vi "Direttore.vi"() -> ()   [LabVIEW 2012]
uses:
  <vilib>/Platform/TimedLoop/XDataNode/timing_clust.ctl
  <vilib>/Platform/TimedLoop/XDataNode/nitl_modes.ctl
  <vilib>/Platform/TimedLoop/XDataNode/wakeup.ctl
  <vilib>/FPGAPlugInAG/PCIe-7852R/niLvFpga_Open_PCIe-7852R.vi
  <vilib>/rvi/interface/common/dynamic/niFpgaDynamicAddResources.vi
  <vilib>/FPGAPlugInAG/Dynamic/niLvFpga_Run_Dynamic.vi
  <vilib>/Utility/error.llb/Error Cluster From Error Code.vi
  <vilib>/rvi/errors/niLvFpgaAdjustHostInterfaceError.vi
  <vilib>/FPGAPlugInAG/Dynamic/niLvFpga_Abort_Dynamic.vi
  <vilib>/FPGAPlugInAG/Dynamic/niLvFpga_Close_Dynamic.vi
  <vilib>/rvi/interface/nirviOpenFPGA/nirviOpenFPGA.xnode
  FPGA Bitfiles/Direttore.lvbitx
  FPGA/Direttore.fpga.vi
  <vilib>/rvi/interface/nirviMethod/nirviMethod.xnode
  <vilib>/Platform/TimedLoop/XDataNode/XDataNode.xnode
  <vilib>/rvi/interface/nirviCloseFPGA/nirviCloseFPGA.xnode
  <vilib>/rvi/errors/niLvFpgaMergeErrorWithErrorCode.vi
  <vilib>/FPGAPlugInAG/Dynamic/niLvFpga_WriteFifo_Dynamic.vi
  <vilib>/FPGAPlugInAG/Dynamic/niLvFpga_ConfigureFifo_Dynamic.vi
  <vilib>/Analysis/NI_AALPro.lvlib
  <vilib>/Platform/TimedLoop/XDataNode/XDNodeRunTimeDep.lvlib
panel:
  out "Matrix (out)":i16[](graph)
  in  "readout channel":i32
  out "Iteration Duration":i64
  in  "duration":dbl=1.0 format="%0.2f"
  in  "square wave duty cycle (%)":dbl=50.0 format="%0.2f"
  in  "phase in":dbl format="%0.2f"
  in  "signal type":T1(ring)
  out "Finished Late? [i-1]":bool
  in  "stop":bool
  out "iterations":i32
  in  "command":i32=1
  in  "dc offset":dbl format="%0.2f"
  in  "amplitude":i16=1
  in  "frequency":dbl=10.0 format="%0.2f"
  out "Empty Elements Remaining trigger FIFO":u32
  out "Empty Elements Remaining OutPutMatrix FIFO":u32
  out "update time":u32
  out "Actual Depth 2":u32
  out "Actual Depth":u32
  out "error out":errorcluster
  in  "error in":errorcluster
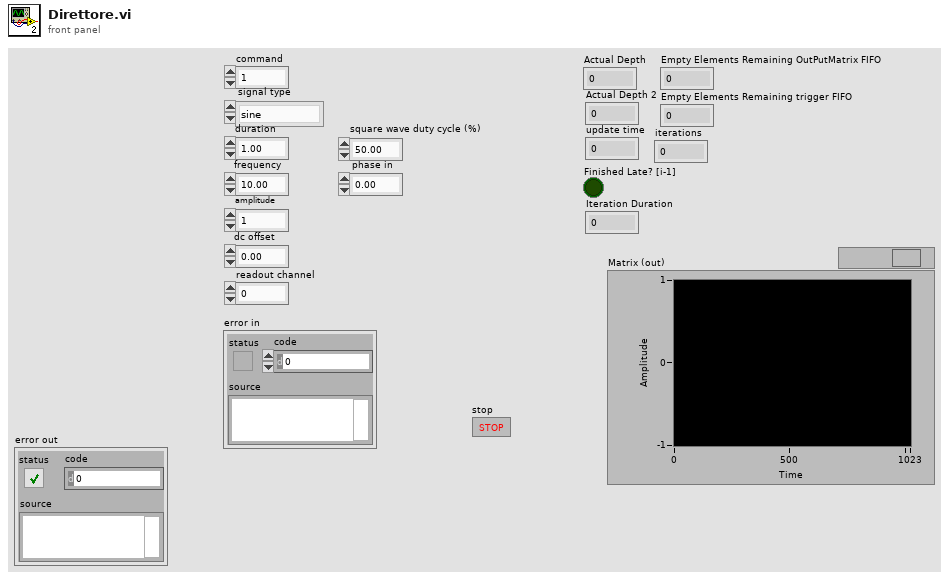
[diagram p1: front panel]
types:
  T1 = enum16{"sine", "cosine", "triangle", "square", "sawtooth", "increasing ramp", "decreasing ramp"}
  T2 = typedef "XDNodeRunTimeDep.lvlib/timing_clust.ctl" = cluster{"Expected End [f-1]":u64, "Actual End [f-1]":u64, "Finished Late? [f-1]":bool, "Expected End [i-1]":u64, "Actual End [i-1]":u64, "Finished Late? [i-1]":bool, "Expected Start [i]":u64, "Actual Start [i]":u64, "Expected Start [f]":u64, "Actual Start [f]":u64, "Source Name":string, "Structure Name":string, "Period":i64, "Deadline":i64, "Offset":i64, "Start":i64, "Priority":i32, "Timeout":i32, "Mode":T3, "Wakeup Reason":T4, "Error":errorcluster, "Source Type":string, "Secondary Source Type":string, "Global End Time":u64, "Global Start Time":u64, "Frame Duration":u64, "Iteration Duration":u64, "Assigned CPU":i32, "I/O Scan Engine Mode":u32}
  T3 = typedef "XDNodeRunTimeDep.lvlib/nitl_modes.ctl" = enum32{"No Change", "Process missed periods, maintain original phase", "Discard missed periods, maintain original phase", "Process missed periods, ignore original phase", "Discard missed periods, ignore original phase"}
  T4 = typedef "XDNodeRunTimeDep.lvlib/wakeup.ctl" = enum32{"Normal", "Aborted", "Asynchronous wakeup", "Timing source error", "Timed loop error", "Timeout"}
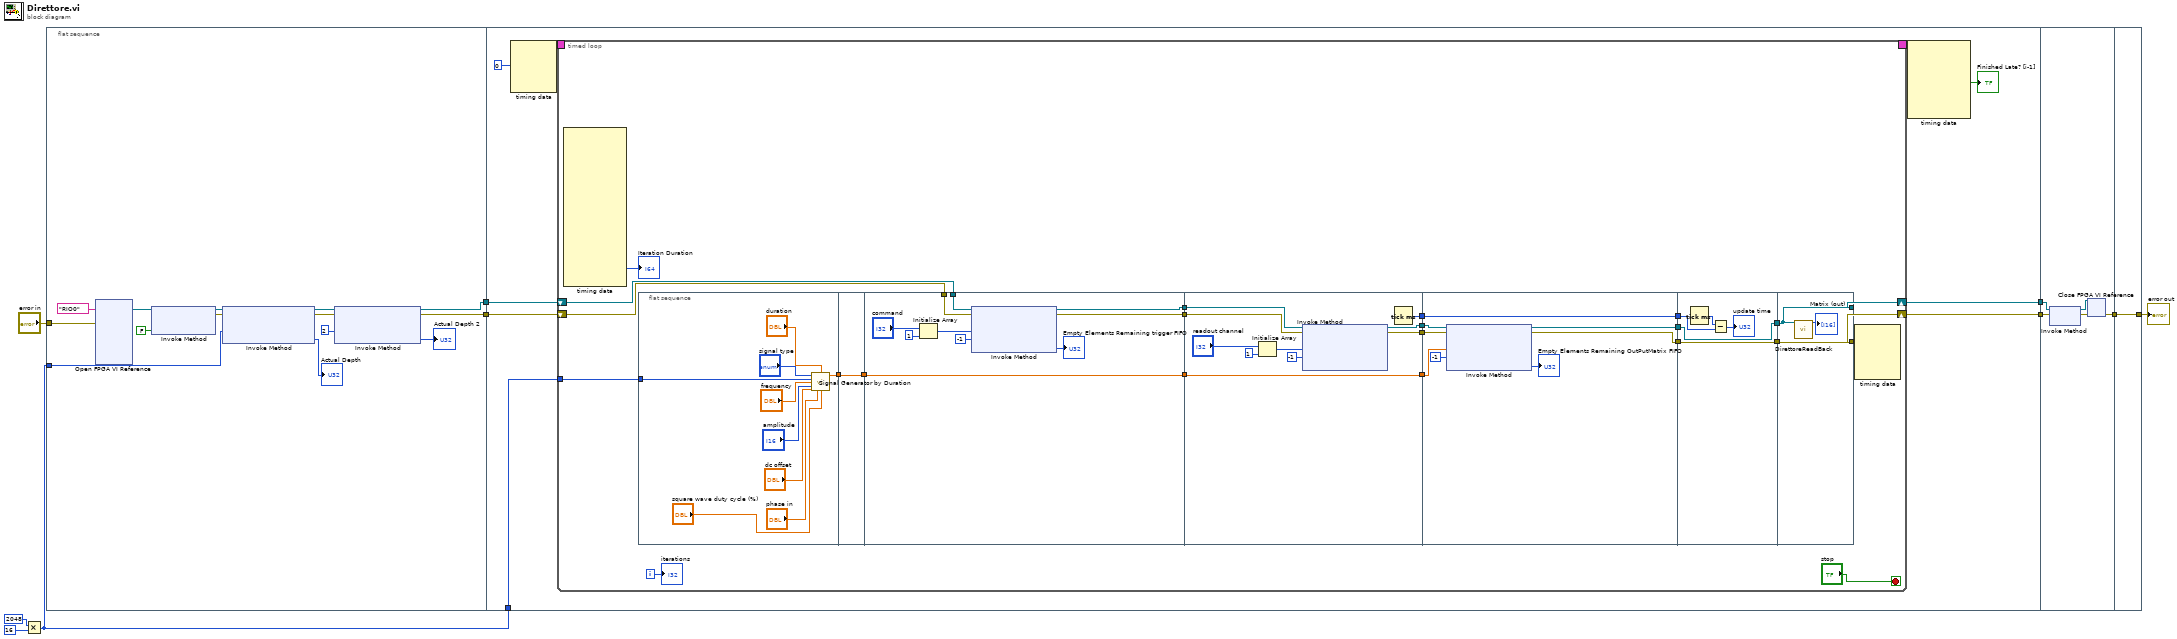
[diagram p0: block diagram]
diagram:
  n1 = Multiply(x=2048 ("Requested Depth"), y=16) -> (x*y=w2:i32)
  n2 = flat-sequence {
    tunnel: "error in" -> [w24]
    tunnel: w2 -> [w14]
    tunnel: [w13] -> w7
    tunnel: [w12] -> w6
    tunnel: w7 -> [w33]
    tunnel: w6 -> [w32]
    tunnel: w2 -> [w31]
    tunnel: [w30] -> w5
    tunnel: [w29] -> w4
    tunnel: [w112] -> w8
    tunnel: w5 -> [w111]
    tunnel: w4 -> [w110]
    tunnel: [w115] -> w9
    tunnel: w8 -> [w115]
    frame #0 {
      n3 = xnode "Open FPGA VI Reference"("error in"=w24, "resource name"=tag "RIO0") -> ("FPGA VI Reference Out"=w22:refnum<k20>)  [unwired: 1 out]
      n4 = xnode "Invoke Method"("FPGA VI Reference In"=w22, "Wait Until Done (F)"=FALSE) -> ("FPGA VI Reference Out"=w21:refnum<k20>, "error out"=w20:errorcluster)  [unwired: 1 in]
      n5 = xnode "Invoke Method"("FPGA VI Reference In"=w21, "error in"=w20, "Requested Depth"=w14) -> ("FPGA VI Reference Out"=w18:refnum<k20>, "error out"=w17:errorcluster, "Actual Depth"=→"Actual Depth":u32)
      n6 = xnode "Invoke Method"("FPGA VI Reference In"=w18, "error in"=w17, "Requested Depth"=u32 2) -> ("FPGA VI Reference Out"=w13:refnum<k20>, "error out"=w12:errorcluster, "Actual Depth"=→"Actual Depth 2":u32)
    }
    frame #1 {
      n7 = node-c288(i64 0 ("Period")) -> (w28:T2)  [unwired: 3 in]
      n8 = timed-loop {
        tunnel: w31 -> [w51]
        shift-right: [w48] -> w30
        shift-left: w33 -> [w53]
        shift-right: [w46] -> w29
        shift-left: w32 -> [w52]
        timing: w28 -> [_]
        timing-out: [_] -> w27
        i -> [w50]
        stop <- "stop" stop-if-true
        n9 = node-c288() -> (→"Iteration Duration":i64)  [unwired: 1 in, 16 out]
        n10 = flat-sequence {
          tunnel: [w67] -> w54
          tunnel: w51 -> [w66]
          tunnel: [w68] -> w55
          tunnel: w54 -> [w68]
          tunnel: w55 -> [w69]
          tunnel: w53 -> [w75]
          tunnel: w52 -> [w74]
          tunnel: [w73] -> w42
          tunnel: [w72] -> w40
          tunnel: [w69] -> w39
          tunnel: w42 -> [w83]
          tunnel: [w84] -> w41
          tunnel: w40 -> [w86]
          tunnel: w39 -> [w88]
          tunnel: [w88] -> w38
          tunnel: [w87] -> w37
          tunnel: [w85] -> w36
          tunnel: w41 -> [w94]
          tunnel: [w92] -> w47
          tunnel: [w91] -> w45
          tunnel: w38 -> [w90]
          tunnel: [w89] -> w44
          tunnel: w37 -> [w89]
          tunnel: w36 -> [w93]
          tunnel: w47 -> [w99]
          tunnel: w45 -> [w98]
          tunnel: w44 -> [w97]
          tunnel: [w99] -> w35
          tunnel: [w98] -> w34
          tunnel: [w104] -> w46
          tunnel: [w103] -> w48
          tunnel: w35 -> [w103]
          tunnel: w34 -> [w104]
          frame #0 {
            n11 = call <vilib>:"Signal Generator by Duration.vi"("signal type"="signal type", "duration"="duration", "# of samples"=w66, "frequency"="frequency", "amplitude"="amplitude", "dc offset"="dc offset", "phase in"="phase in", "square wave duty cycle (%)"="square wave duty cycle (%)") -> ("signal"=w67:dbl[])  [unwired: 4 in, 3 out]
          }
          frame #1 {
          }
          frame #2 {
            n12 = Initialize Array("command", 1 ("dimension size")) -> (w76:i32[])
            n13 = xnode "Invoke Method"("FPGA VI Reference In"=w75, "error in"=w74, "Data"=w76, "Timeout (ms)"=-1) -> ("FPGA VI Reference Out"=w73:refnum<k20>, "error out"=w72:errorcluster, "Empty Elements Remaining"=→"Empty Elements Remaining trigger FIFO":u32)
          }
          frame #3 {
            n14 = Initialize Array("readout channel", 1 ("dimension size")) -> (w79:i32[])
            n15 = xnode "Invoke Method"("FPGA VI Reference In"=w83, "error in"=w86, "Data"=w79, "Timeout (ms)"=-1) -> ("FPGA VI Reference Out"=w84:refnum<k20>, "error out"=w85:errorcluster)  [unwired: 1 out]
            n16 = Tick Count (ms)() -> (millisecond timer value=w87:u32)
          }
          frame #4 {
            n17 = xnode "Invoke Method"("FPGA VI Reference In"=w94, "error in"=w93, "Data"=w90, "Timeout (ms)"=-1) -> ("FPGA VI Reference Out"=w92:refnum<k20>, "error out"=w91:errorcluster, "Empty Elements Remaining"=→"Empty Elements Remaining OutPutMatrix FIFO":u32)
          }
          frame #5 {
            n18 = Tick Count (ms)() -> (millisecond timer value=w100:u32)
            n19 = Subtract(x=w100, y=w97) -> (x-y=→"update time":u32)
          }
          frame #6 {
            n20 = call "DirettoreReadBack.vi"("FPGA VI Reference (in)"=w103) -> ("Matrix (out)"=→"Matrix (out)":i16[])  [unwired: 13 in, 1 out]
          }
        }
        n21 = node-c288() -> ()  [unwired: 5 in, 1 out]
        "iterations" <- w50
      }
      n22 = node-c288(w27) -> (→"Finished Late? [i-1]":bool)  [unwired: 6 out]
    }
    frame #2 {
      n23 = xnode "Invoke Method"("FPGA VI Reference In"=w111, "error in"=w110) -> ("FPGA VI Reference Out"=w114:refnum<k20>, "error out"=w113:errorcluster)
      n24 = xnode "Close FPGA VI Reference"("FPGA VI Reference In"=w114, "error in"=w113) -> ("error out"=w112:errorcluster)
    }
    frame #3 {
    }
  }
  "error out" <- w9
